vi "assignment2b.vi"() -> ()   [LabVIEW 2021]
panel:
  out "Surveillance camera":bool
  in  "?":bool
  out "Time loading":u8(slide) scale=0.0..100.0
  in  "?":bool
  out "System movement controller":bool
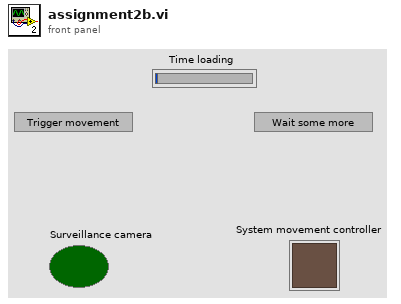
[diagram p1: front panel]
types:
  T1 = enum16{"PromtQuestion", "Wait", "RequestAnswear", "Done"}
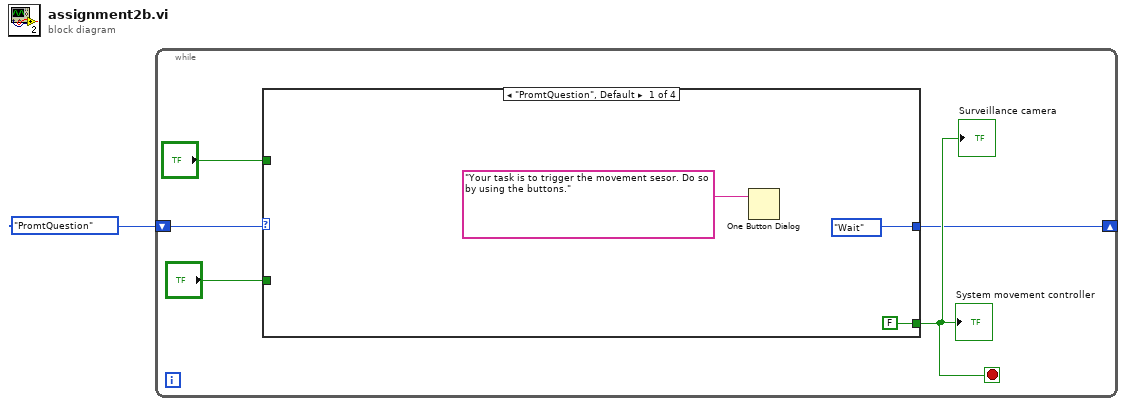
[diagram p0: block diagram]
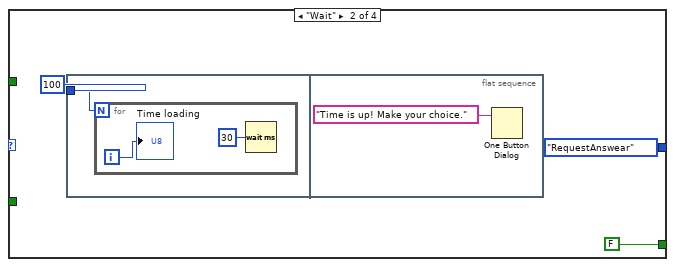
[diagram p2: hidden frame]
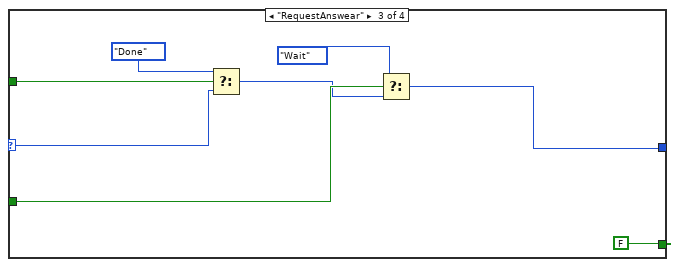
[diagram p3: hidden frame]
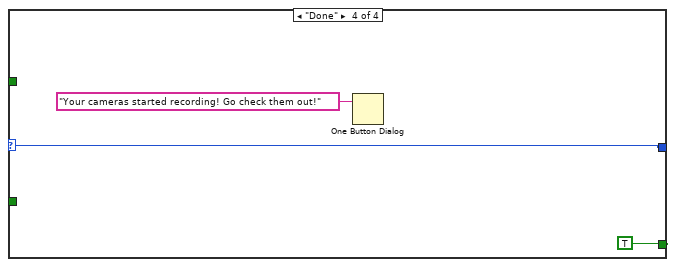
[diagram p4: hidden frame]
diagram:
  n1 = while {
    shift-right: [w2] -> _
    shift-left: T1."PromtQuestion" -> [w6]
    stop <- w3 stop-if-true
    n2 = case shown="\"PromtQuestion\", Default" w6 {
      selector: w6 -> [_ _ w22 w25]
      tunnel: [FALSE FALSE FALSE TRUE] -> w3
      tunnel: "?" -> [_ _ w24 _]
      tunnel: "?" -> [_ _ w21 _]
      tunnel: [T1."Wait" T1."RequestAnswear" w17 w25] -> w2
      frame "PromtQuestion", Default {
        n3 = One Button Dialog(message="Your task is to trigger the movement sesor. Do so by using the buttons.") -> ()  [unwired: 1 in, 1 out]
      }
      frame "Wait" {
        n4 = flat-sequence {
          tunnel: 100 -> [w13]
          frame #0 {
            n5 = for {
              N: w13 -> [_]
              i -> [w14]
              n6 = Wait (ms)(milliseconds to wait=u32 30) -> ()  [unwired: 1 out]
              "Time loading" <- w14
            }
          }
          frame #1 {
            n7 = One Button Dialog(message="Time is up! Make your choice." ("Teacher is thinking!")) -> ()  [unwired: 1 in, 1 out]
          }
        }
      }
      frame "RequestAnswear" {
        n8 = Select(t=T1."Done", s=w24, f=w22) -> (s? t:f=w20:T1)
        n9 = Select(t=T1."Wait", s=w21, f=w20) -> (s? t:f=w17:T1)
      }
      frame "Done" {
        n10 = One Button Dialog(message="Your cameras started recording! Go check them out!") -> ()  [unwired: 1 in, 1 out]
      }
    }
    "System movement controller" <- w3
    "Surveillance camera" <- w3
  }
